vi "Mutex Timed Lock (relative nanoseconds).vi"(8 "error in (no error)":errorcluster, 10 "relative timeout (nanoseconds)":i64, 11 "Mutex in":T1) -> (0 "error out":errorcluster, 2 "timed out?":bool, 3 "Mutex out":T1)   [LabVIEW 2013, in "POSIX Threads.lvlib" / "Mutex.lvclass"]
doc: "Calls pthread_mutex_timedlock() on the pthread mutex object encapsulated by Mutex.\n\nThis VI attempts to lock the provided mutex in a specified timeout period.\n\nRefer to online POSIX documentation for more information."
uses:
  Mutex.lvclass
  Controls/reference.ctl
  <vilib>/NI/NI Linux RT Utilities/Controls/Public/C Enums/clockid_t.ctl
  POSIX Thread Object/POSIX Thread Object.lvclass/POSIX Thread Object.ctl
  POSIX Thread Object/Private VIs/libpthread path.vi
  <vilib>/NI/NI Linux RT Utilities/VIs/Public/Convert Types/convert timespec 64 to timespec 32.vi
  <vilib>/NI/NI Linux RT Utilities/VIs/Public/Time/Increment Time (timespec).vi
  <vilib>/NI/NI Linux RT Utilities/VIs/Public/Time/Get Clock Time (timespec).vi
  POSIX Thread Object/Private VIs/get pthread error.vi
  POSIX Thread Object/POSIX Thread Object.lvclass
  <vilib>/NI/NI Linux RT Utilities/Linux RT Utilities.lvlib
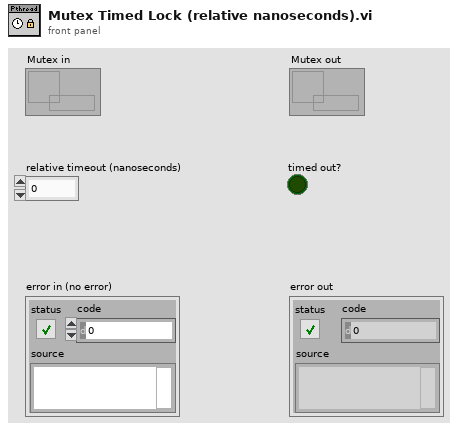
[diagram p1: front panel]
types:
  T1 = typedef "POSIX Threads.lvlib/Mutex.lvclass/reference.ctl" = refnum<data-value>
  T2 = typedef "Linux RT Utilities.lvlib/clockid_t.ctl" = enum16{"Realtime", "Monotonic"}
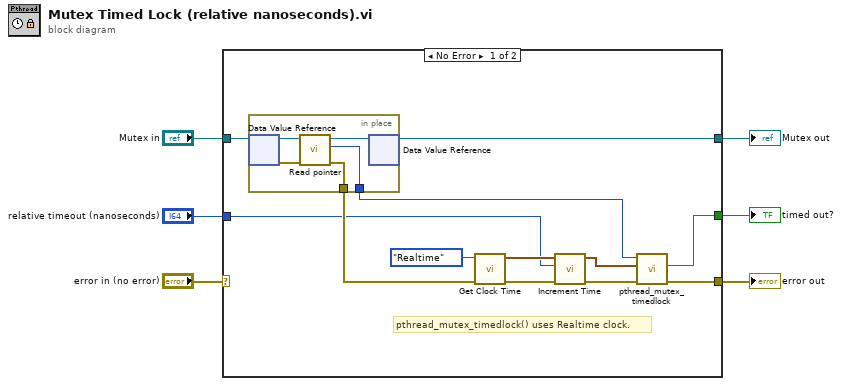
[diagram p0: block diagram]
diagram:
  n1 = case shown="No Error" "error in (no error)" {
    selector: "error in (no error)" -> [_ w25]
    tunnel: [w18 w25] -> w5
    tunnel: "Mutex in" -> [w11 w24]
    tunnel: [w10 w24] -> w3
    tunnel: "relative timeout (nanoseconds)" -> [w8 _]
    tunnel: [w17 _] -> w1
    frame No Error {
      # "pthread_mutex_timedlock() uses Realtime clock."
      n2 = in-place {
        in-place-border: [w20] -> w9
        in-place-border: [w19] -> w7
        n3 = in-place-dvr #1(w11) -> (w23:refnum<class "Mutex.lvclass">, w21:errorcluster)
        n4 = call "Read pointer.vi"("error in (no error)"=w21, "POSIX Thread Object in"=w23) -> ("error out"=w20:errorcluster, "pointer"=w19:u64, "POSIX Thread Object out"=w22:refnum<class "Mutex.lvclass">)  [unwired: 7 in]
        n5 = in-place-dvr #1(w22) -> (w10:T1)  [unwired: 1 out]
      }
      n6 = call-poly <vilib>:"Get Clock Time.vi"("error in (no error)"=w9, "clock id (realtime)"=clockid_t."Realtime" ("clock id (monotonic)")) -> ("error out"=w15:errorcluster, "timespec"=w13:cluster{"sec":u64, "nsec":u64})  [unwired: 8 in]
      n7 = call-poly <vilib>:"Increment Time.vi"("error in (no error)"=w15, "nanoseconds to add"=w8, "timespec in"=w13) -> ("error out"=w16:errorcluster, "timespec out"=w12:cluster{"sec":u64, "nsec":u64})  [unwired: 7 in]
      n8 = call "pthread_mutex_timedlock.vi"("error in (no error)"=w16, "absolute time"=w12, "mutex ptr in"=w7) -> ("error out"=w18:errorcluster, "timed out?"=w17:bool)  [unwired: 6 in, 1 out]
    }
    frame Error {
    }
  }
  "Mutex out" <- w3
  "error out" <- w5
  "timed out?" <- w1
